vi "Cepillo_Lavado.vi"() -> ()   [LabVIEW 2020]
panel:
  out "Cepillo lavado":bool
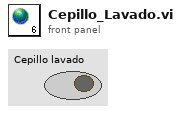
[diagram p1: front panel]
diagram:
